vi "ATF Storage-DI_Read.vi"(7 "number of samples per channel":i32, 8 "error in (no error)":errorcluster, 10 "Data FIFO Ref":T1, 11 "DI_Task":refnum<k21>) -> (0 "error out":errorcluster, 3 "task out":refnum<k21>)   [LabVIEW 2022 SP3]
uses:
  RT Controls/ATF Storage-Data FIFO.ctl
  RT Controls/ATF Storage Haelth.ctl
  <vilib>/DAQmx/read.llb/DAQmx Read (Digital 1D Wfm NChan NSamp).vi
  <vilib>/DAQmx/miscellaneous.llb/DAQmx Fill In Error Info.vi
  RT Support/ATF Storage-RT_Global_R.vi
panel:
  out "overflow?":bool
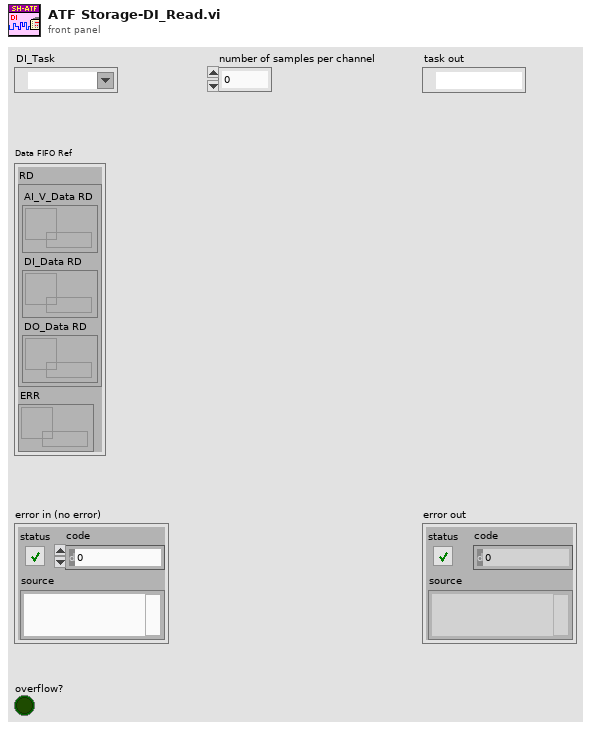
[diagram p1: front panel]
types:
  T1 = typedef "ATF Storage-Data FIFO.ctl" = cluster{"RD":cluster{"AI_V_Data RD":refnum<queue>, "DI_Data RD":refnum<queue>, "DO_Data RD":refnum<queue>}, "ERR":refnum<queue>}
  T2 = typedef "ATF Storage Haelth.ctl" = enum16{"AI C", "AI V", "AO", "DI", "DO", "TC", "ACC", "RT Str", "DR A"}
  T3 = enum16{"Init", "Read 'All'", "Read 'n'", "Read '1'", "Write '1'", "Write 'n'", "Write 'All'"}
  T4 = cluster{"Start DAQ":bool, "Stop DAQ":bool, "RT Stop":bool, "RT Exit":bool, "Start Seq":bool}
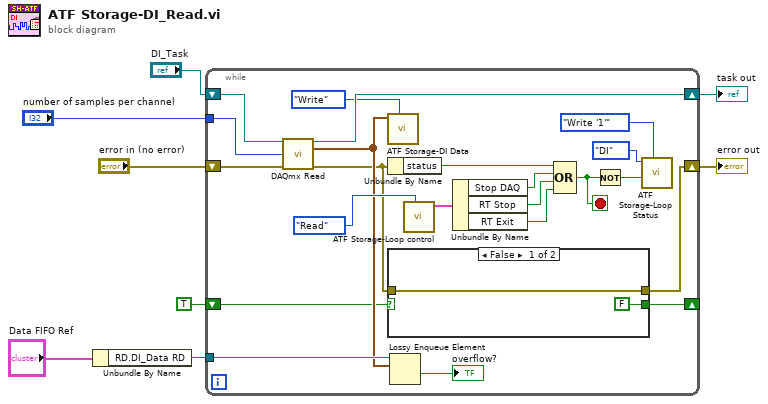
[diagram p0: block diagram]
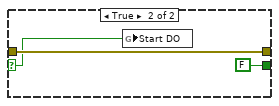
[diagram p2: hidden frame]
diagram:
  n1 = Unbundle By Name("Data FIFO Ref") -> ("RD.DI_Data RD"=w2:refnum<queue>)
  n2 = while {
    tunnel: "number of samples per channel" -> [w15]
    tunnel: w2 -> [w18]
    shift-right: [w19] -> w5
    shift-left: "DI_Task" -> [w29]
    shift-right: [w9] -> w4
    shift-left: "error in (no error)" -> [w28]
    shift-right: [w11] -> _
    shift-left: TRUE -> [w12]
    stop <- w30 stop-if-true
    n3 = call-poly <vilib>:"DAQmx Read.vi"("task/channels in"=w29, "number of samples per channel"=w15, "error in"=w28) -> ("task out"=w19:refnum<k21>, "data"=w13:digitalwaveform[], "error out"=w10:errorcluster)  [unwired: 10 in]
    n4 = call "ATF Storage-DI Data.vi"("Enum"=enum16{"Write", "Read"}."Write", "In_DI data"=w13) -> ()  [unwired: 9 in, 1 out]
    n5 = Unbundle By Name(w10) -> ("status"=w27:bool)
    n6 = case shown="False" w12 {
      selector: w12 -> [_ w33]
      tunnel: [FALSE FALSE] -> w11
      tunnel: w10 -> [w31 w34]
      tunnel: [w31 w34] -> w9
      frame False {
      }
      frame True {
        n7 = global write "ATF Storage-RT_Global_R.vi" "Start DO"(w33) -> ()
      }
    }
    n8 = Lossy Enqueue Element(queue=w18, element=w13) -> (overflow?=→"overflow?":bool)  [unwired: 1 in, 3 out]
    n9 = call "ATF Storage-Loop control.vi"("Action"=enum16{"Init", "Write", "Read"}."Read") -> ("Loop Control out"=w22:T4)  [unwired: 9 in, 1 out]
    n10 = Unbundle By Name(w22) -> ("Stop DAQ"=w26:bool, "RT Stop"=w25:bool, "RT Exit"=w24:bool)
    n11 = Compound Arithmetic op=OR(w27, w26, w25, w24) -> (w30:bool)
    n12 = Not(x=w30) -> (.not. x?=w20:bool)
    n13 = call "ATF Storage-Loop Status.vi"("Option"=T3."Write '1'", "Status"=w20, "Loop"=ATF_Storage_Haelth."DI") -> ()  [unwired: 6 in, 3 out]
  }
  "task out" <- w5
  "error out" <- w4
